vi "ShooterConfig.vi"(6 "Auto in":bool=TRUE, 7 "Mode":T1=enum."Read", 8 "error in (no error)":errorcluster, 9 "Reset After Fire In":bool=TRUE, 10 "Full Reset In":bool=TRUE, 11 "Fire After Retract Full In":bool=TRUE) -> (0 "error out":errorcluster, 1 "Reset After Fire":bool, 2 "Full Reset":bool, 3 "Fire After Retract Full":bool, 4 "Auto":bool)   [LabVIEW 2013]
uses:
  ShooterConfigModes.ctl
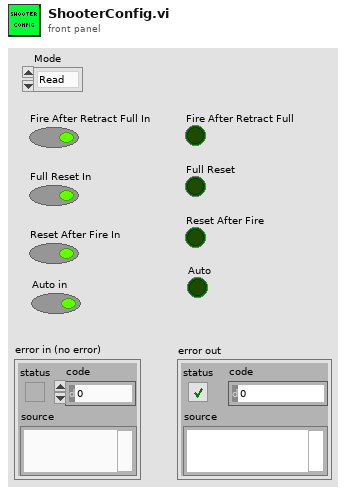
[diagram p1: front panel]
types:
  T1 = typedef "ShooterConfigModes.ctl" = enum16{"Init", "Read", "Set All", "Set Fire After Retract Full"}
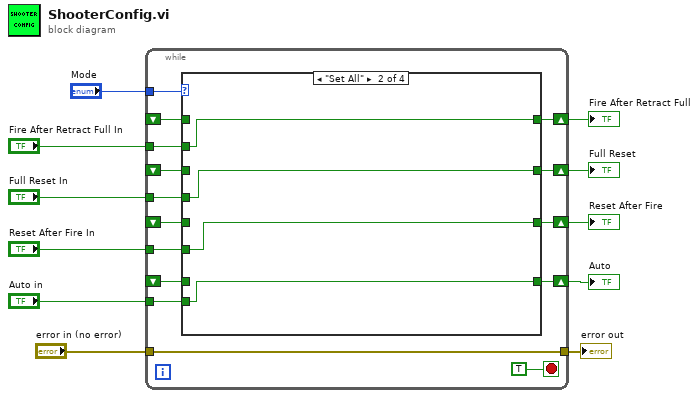
[diagram p0: block diagram]
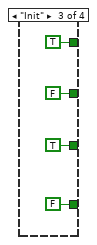
[diagram p3: hidden frame]
diagram:
  n1 = while {
    tunnel: "Mode" -> [w25]
    tunnel: "Fire After Retract Full In" -> [w24]
    shift-right: [w23] -> w6
    shift-left: _ -> [w22]
    tunnel: "Full Reset In" -> [w19]
    shift-right: [w20] -> w7
    shift-left: _ -> [w21]
    tunnel: "Reset After Fire In" -> [w18]
    shift-right: [w17] -> w10
    shift-left: _ -> [w16]
    tunnel: "error in (no error)" -> [w15]
    tunnel: [w15] -> w3
    tunnel: "Auto in" -> [w14]
    shift-right: [w13] -> w1
    shift-left: _ -> [w12]
    stop <- TRUE stop-if-true
    n2 = case shown="\"Set All\"" w25 {
      tunnel: w24 -> [_ w34 _ w42]
      tunnel: [w30 w34 TRUE ("Fire After Retract Full In") w42] -> w23
      tunnel: w22 -> [w30 _ _ _]
      tunnel: w19 -> [_ w33 _ _]
      tunnel: [w29 w33 FALSE ("Full Reset In") w41] -> w20
      tunnel: w21 -> [w29 _ _ w41]
      tunnel: w18 -> [_ w32 _ _]
      tunnel: [w28 w32 TRUE ("Reset After Fire In") w40] -> w17
      tunnel: w16 -> [w28 _ _ w40]
      tunnel: w14 -> [_ w31 _ _]
      tunnel: [w27 w31 FALSE ("Auto in") w39] -> w13
      tunnel: w12 -> [w27 _ _ w39]
      frame "Read", Default {
      }
      frame "Set All" {
      }
      frame "Init" {
      }
      frame "Set Fire After Retract Full" {
      }
    }
  }
  "Fire After Retract Full" <- w6
  "Full Reset" <- w7
  "Reset After Fire" <- w10
  "error out" <- w3
  "Auto" <- w1
